vi "Gradient Read Single.vi"(8 "error in":errorcluster, 9 "Channel Index":i32=1, 11 "Humidity Gradient in":refnum<class "Humidity Gradient.lvclass">) -> (0 "error out":errorcluster, 1 "Changed or First Call?":bool, 2 "Humidity SP":dbl, 3 "Humidity Gradient out":refnum<class "Humidity Gradient.lvclass">)   [LabVIEW 2023, in "Humidity Gradient.lvclass"]
uses:
  Humidity Gradient.lvclass
  Parents/Gradient/Gradient.lvclass
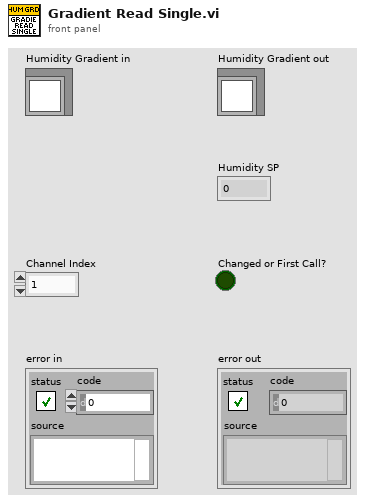
[diagram p1: front panel]
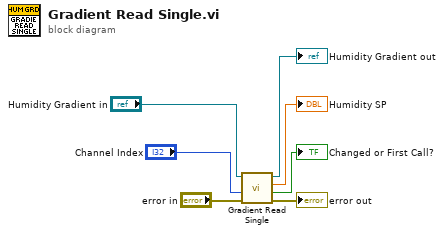
[diagram p0: block diagram]
diagram:
  n1 = call-parent "Gradient Read Single.vi"("error in"="error in", "Channel Index"="Channel Index", "Gradient in"="Humidity Gradient in") -> ("error out"=→"error out":errorcluster, "Changed or First Call?"=→"Changed or First Call?":bool, "Current SP"=→"Humidity SP":dbl, "Gradient out"=→"Humidity Gradient out":refnum<class "Humidity Gradient.lvclass">)  [unwired: 5 in]
